vi "easy stream start U6.vi"(4 "Advanced":T1={"PC buffer size (seconds)"=10.0, "Resolution Index"=0, "StreamSettlingFactor"=0, "Binary"=FALSE} {"PC buffer size (seconds)" format="%.2f"}, 6 "Scan List (-)":u8[](array[numeric]), 7 "Device Info":T2={"DeviceType"=6, "Connection Type"=0, "Address"="1", "FirstFound"=TRUE} {"Connection Type" items=["USB", "Ethernet"]}, 8 "error in":errorcluster, 9 "Scan List (+)":u8[](array[numeric])=[0, 1, 2, 3], 10 "Scan Rate (Hz)":dbl=1000.0 format="%.3f", 11 "Range Constants":u8[](array[ring]) items=["LJ_rgBIP10V", "LJ_rgBIP1V", "LJ_rgBIPP1V", "LJ_rgBIPP01V"]) -> (0 "error out":errorcluster, 1 "# Channels":i32, 2 "Actual Scan Rate (Hz)":dbl=1000.0 format="%.3f", 3 "Handle Out":i32)   [LabVIEW 2020]
panel:
  # "By default, this VI configures the\ndevice for \"SLEEP\" stream read wait mode.\n\nScan List (-) only needed if doing something\nbesides single-ended channels.  Ranges array\nonly needed if you want something besides\n+/-10 volts."
  # "3 = U3\n6 = U6\n9 = UE9"
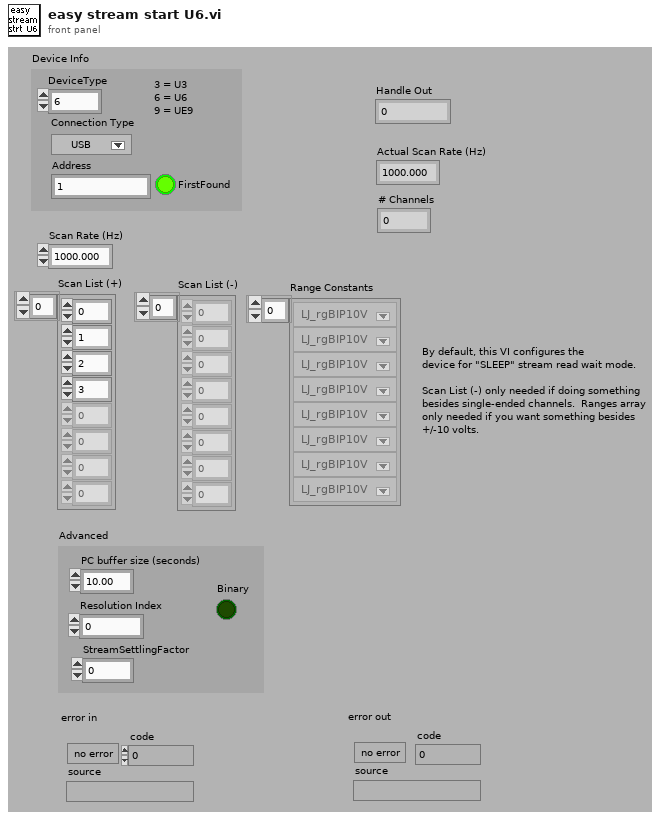
[diagram p1: front panel]
types:
  T1 = cluster{"PC buffer size (seconds)":dbl, "Resolution Index":u8, "StreamSettlingFactor":i32, "Binary":bool}
  T2 = cluster{"DeviceType":i32, "Connection Type":u16, "Address":string, "FirstFound":bool}
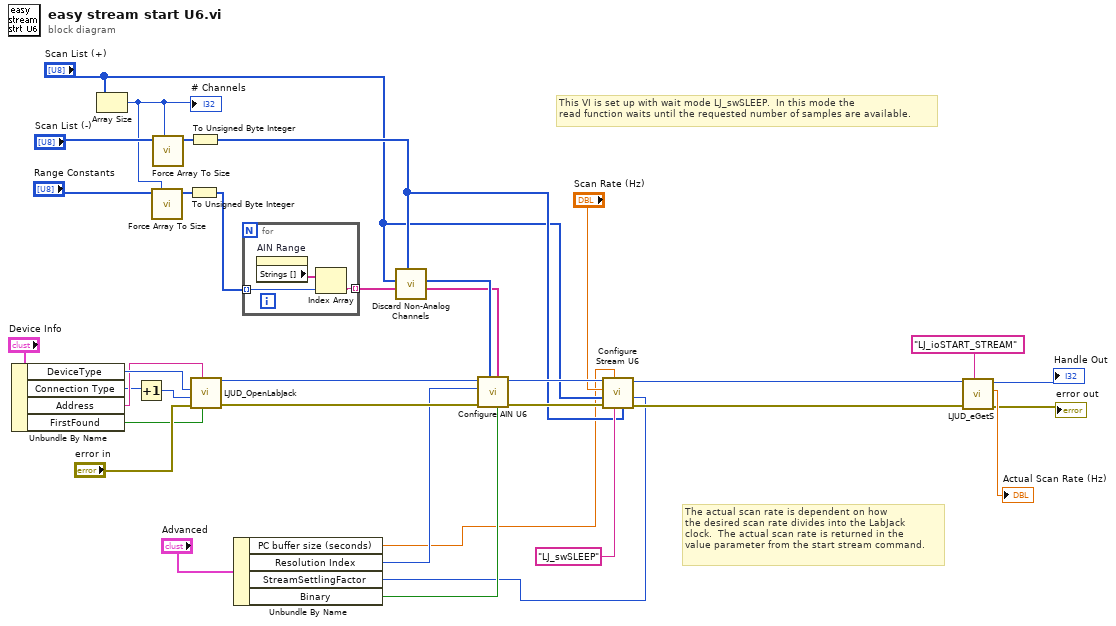
[diagram p0: block diagram]
diagram:
  # "This VI is set up with wait mode LJ_swSLEEP.  In this mode the\nread function waits until the requested number of samples are available."
  # "The actual scan rate is dependent on how\nthe desired scan rate divides into the LabJack\nclock.  The actual scan rate is returned in the\nvalue parameter from the start stream command."
  n1 = Unbundle By Name("Device Info") -> ("DeviceType"=w30:i32, "Connection Type"=w26:u16, "Address"=w28:string, "FirstFound"=w27:bool)
  n2 = Array Size(array="Scan List (+)") -> (size(s)=w8:i32)
  "# Channels" <- w8
  n3 = Increment(x=w26) -> (x+1=w25:u16)
  n4 = call "Force Array To Size.vi"("# Elements"=w8, "I32 Array In"="Range Constants") -> ("I32 Array Out"=w11:i32[])  [unwired: 6 in, 3 out]
  n5 = call "Force Array To Size.vi"("# Elements"=w8, "I32 Array In"="Scan List (-)") -> ("I32 Array Out"=w12:i32[])  [unwired: 6 in, 3 out]
  n6 = To Unsigned Byte Integer(number=w11) -> (unsigned 8bit integer=w2:u8[])
  n7 = To Unsigned Byte Integer(number=w12) -> (unsigned 8bit integer=w10:u8[])
  n8 = call "LJUD_OpenLabJack.vi"("FirstFound"=w27, "Address"=w28, "error in"="error in", "ConnectionType"=w25, "DeviceType"=w30) -> ("error out"=w19:errorcluster, "Handle"=w18:i32)  [unwired: 5 in]
  n9 = Unbundle By Name("Advanced") -> ("PC buffer size (seconds)"=w4:dbl, "Resolution Index"=w6:u8, "StreamSettlingFactor"=w3:i32, "Binary"=w5:bool)
  n10 = for {
    tunnel: w2 -> [w38] mode=indexing
    tunnel: [w37] -> w1 mode=indexing
    n11 = property on="AIN Range" class="Ring (strict)"() -> ("Strings []"=w36:string[])  [unwired: 2 in, 2 out]
    n12 = Index Array(array=w36, index=w38) -> (element=w37:string)
  }
  n13 = call "Discard Non-Analog Channels.vi"("Channels In (-)"=w10, "Ranges In"=w1, "Channels In"="Scan List (+)") -> ("Ranges Out"=w20:string[], "Channels Out"=w21:i32[])  [unwired: 5 in, 2 out]
  n14 = call "Configure AIN U6.vi"("Binary"=w5, "Ranges"=w20, "Positive Channels"=w21, "error in"=w19, "Resolution"=w6, "Handle In"=w18) -> ("error out"=w23:errorcluster, "Handle Out"=w22:i32)  [unwired: 4 in]
  n15 = call "Configure Stream U6.vi"("SettlingFactor"=w3, "Scan List (-)"=w10, "Wait Mode"="LJ_swSLEEP" ("Wait Mode (2)"), "PC buffer size (seconds)"=w4, "error in"=w23, "Scan List (+)"="Scan List (+)", "Scan Rate (Hz)"="Scan Rate (Hz)", "Handle In"=w22) -> ("error out"=w16:errorcluster, "Handle Out"=w17:i32)  [unwired: 1 in, 1 out]
  n16 = call "LJUD_eGetS.vi"("IOType"="LJ_ioSTART_STREAM", "error in"=w16, "Handle In"=w17) -> ("error out"=→"error out":errorcluster, "Value Read"=→"Actual Scan Rate (Hz)":dbl, "Handle Out"=→"Handle Out":i32)  [unwired: 6 in]
